vi "Out_S2F37.vi"(8 "error in (no error)":errorcluster, 10 "S2F37":T1, 11 "S2 Message Class in":refnum<class "S2 Message Class.lvclass">) -> (0 "error out":errorcluster, 3 "S2 Message Class out":refnum<class "S2 Message Class.lvclass">)   [LabVIEW 2020, in "SECS Communication.lvlib" / "S2 Message Class.lvclass"]
uses:
  S2 Message Class.lvclass
  D:/Dropbox/SECS/SECS_GEM v1.0.7/Com/SECS Communication/SECS-II Class/SECS-II Class.lvclass
  S2F37.ctl
  SECS-II Class/Data Message_List.vi
  SECS-II Class/Data Message_Boolean.vi
  SECS-II Class/Data Message_U4.vi
  SECS-II Class/SECS-II Class.lvclass
  D:/Dropbox/SECS/SECS_GEM v1.0.7/Com/SECS Communication/S2 Message Class/S2 Message Class.lvclass
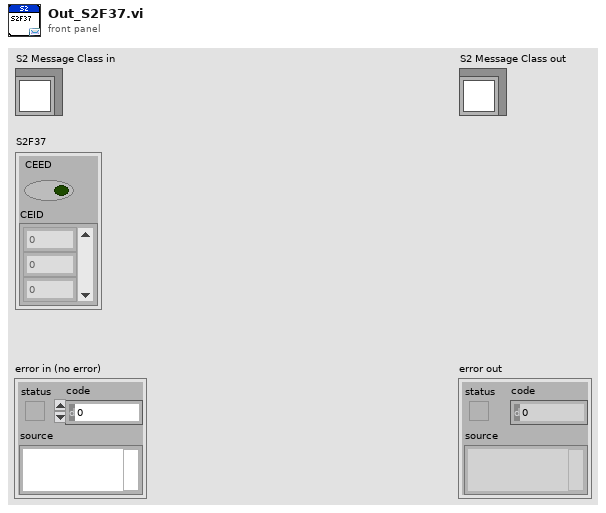
[diagram p1: front panel]
types:
  T1 = typedef "SECS Communication.lvlib/S2 Message Class.lvclass/S2F37.ctl" = cluster{"CEED":bool, "CEID":u32[]}
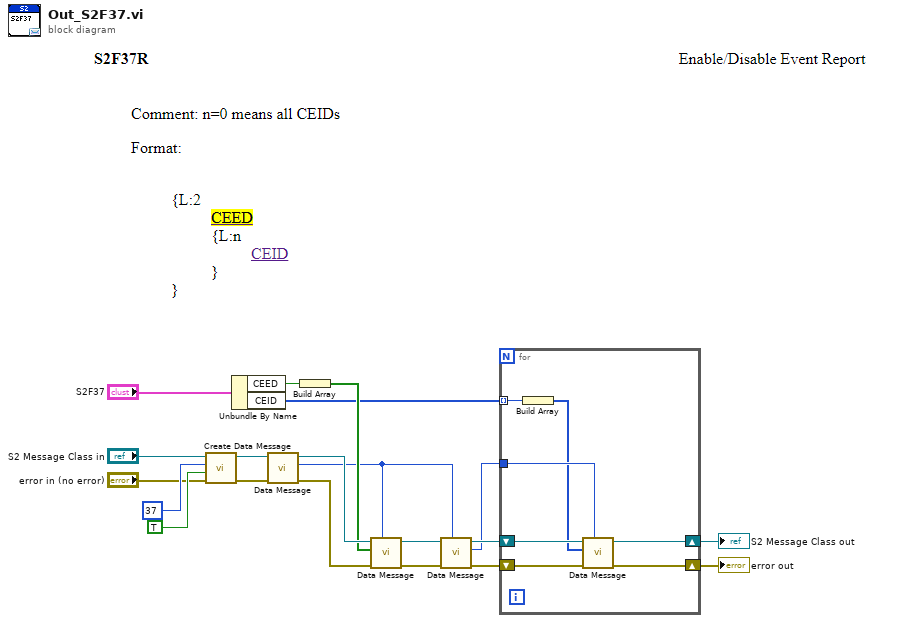
[diagram p0: block diagram]
diagram:
  n1 = call "Create Data Message.vi"("error in (no error)"="error in (no error)", "W-Bit"=TRUE, "Function"=u8 37, "SECS-II Class in"="S2 Message Class in") -> ("error out"=w16:errorcluster, "SECS-II Class out"=w15:refnum<class "S2 Message Class.lvclass">)  [unwired: 6 in]
  n2 = Unbundle By Name("S2F37") -> ("CEED"=w11:bool, "CEID"=w3:u32[])
  n3 = call-poly "Data Message.vi"("error in"=w16, "SECS-II Class in"=w15) -> ("error out"=w14:errorcluster, "Index"=w7:i32, "SECS-II Class out"=w13:refnum<class "S2 Message Class.lvclass">)  [unwired: 7 in]
  n4 = Build Array(w11) -> (w10:bool[])
  n5 = call-poly "Data Message.vi"("Parent Index"=w7, "error in"=w14, "Data"=w10, "SECS-II Class in"=w13) -> ("error out"=w9:errorcluster, "SECS-II Class out"=w8:refnum<class "S2 Message Class.lvclass">)  [unwired: 6 in]
  n6 = call-poly "Data Message.vi"("Parent Index"=w7, "error in"=w9, "SECS-II Class in"=w8) -> ("error out"=w6:errorcluster, "Index"=w4:i32, "SECS-II Class out"=w5:refnum<class "S2 Message Class.lvclass">)  [unwired: 6 in]
  n7 = for {
    shift-right: [w22] -> w1
    shift-left: w6 -> [w27]
    shift-right: [w21] -> w2
    shift-left: w5 -> [w26]
    tunnel: w4 -> [w25]
    tunnel: w3 -> [w24] mode=indexing
    n8 = Build Array(w24) -> (w23:u32[])
    n9 = call-poly "Data Message.vi"("Parent Index"=w25, "error in"=w27, "Data"=w23, "SECS-II Class in"=w26) -> ("error out"=w22:errorcluster, "SECS-II Class out"=w21:refnum<class "S2 Message Class.lvclass">)  [unwired: 6 in]
  }
  "error out" <- w1
  "S2 Message Class out" <- w2
